vi "Test image rotation.vi"() -> ()   [LabVIEW 2022 SP3]
uses:
  Typedefs/Top level controls.ctl
panel:
  in  "R_min":dbl=150.0
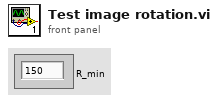
[diagram p1: front panel]
types:
  T1 = typedef "Top level controls.ctl" = cluster{"Auto ROI (for rot.)":bool, "Apply scaling":bool, "Apply rotation":bool, "Apply Tx":bool, "Apply Ty":bool, "Keep proc. img":bool}
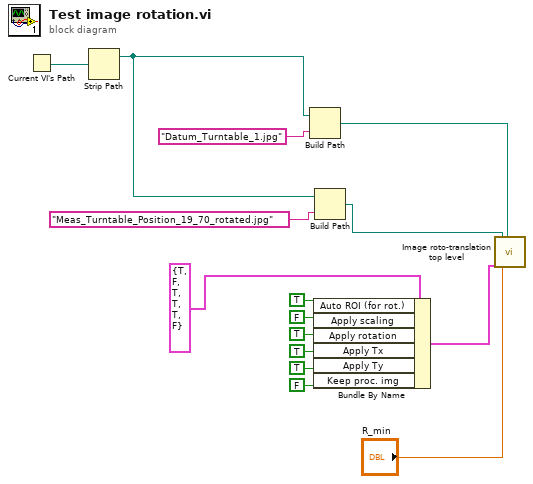
[diagram p0: block diagram]
diagram:
  n1 = Current VI's Path() -> (path=w15:path)
  n2 = Strip Path(path=w15) -> (stripped path=w13:path)  [unwired: 1 out]
  n3 = Build Path(base path=w13, name or relative path="Datum_Turntable_1.jpg") -> (appended path=w11:path)
  n4 = Bundle By Name(cluster=T1 {"Auto ROI (for rot.)"=TRUE, "Apply scaling"=FALSE, "Apply rotation"=TRUE, "Apply Tx"=TRUE, "Apply Ty"=TRUE, "Keep proc. img"=FALSE} ("Controls"), "Auto ROI (for rot.)"=TRUE, "Apply scaling"=FALSE, "Apply rotation"=TRUE, "Apply Tx"=TRUE, "Apply Ty"=TRUE, "Keep proc. img"=FALSE) -> (w8:T1)
  n5 = Build Path(base path=w13, name or relative path="Meas_Turntable_Position_19_70_rotated.jpg") -> (appended path=w10:path)
  n6 = call "Image roto-translation top level.vi"("Controls"=w8, "Test image file path"=w10, "R_min"="R_min", "Reference image file path"=w11) -> ()  [unwired: 8 in, 8 out]
